vi "ReadDispenseCount (SubVI).vi"(10 "Base Path":path) -> (2 "appended array":i32[](array[numeric]))   [LabVIEW 2013]
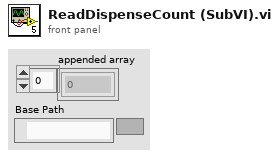
[diagram p1: front panel]
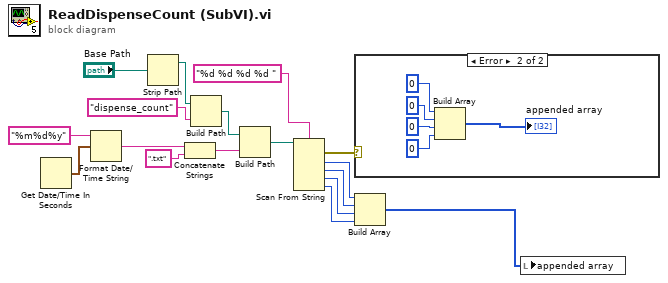
[diagram p0: block diagram]
diagram:
  n1 = Get Date/Time In Seconds() -> (seconds since 1Jan1904=w12:timestamp)
  n2 = Format Date/Time String(time format string (%c)="%m%d%y", seconds (now)=w12) -> (date/time string=w10:string)  [unwired: 1 in]
  n3 = Strip Path(path="Base Path") -> (stripped path=w14:path)  [unwired: 1 out]
  n4 = Concatenate Strings(w10, ".txt" ("string")) -> (w8:string)
  n5 = Build Path(base path=w14, name or relative path="dispense_count") -> (appended path=w17:path)
  n6 = Build Path(base path=w17, name or relative path=w8) -> (appended path=w7:path)
  n7 = Scan From String("%d %d %d %d " ("format string"), w7) -> (w15:errorcluster, output 1=w2:i32, output 2=w5:i32, output 3=w4:i32, output 4=w3:i32)  [unwired: 5 in, 1 out]
  n8 = case shown="Error" w15 {
    frame No Error {
    }
    frame Error {
      n9 = Build Array(0 ("element"), 0 ("element"), 0 ("element"), 0 ("element")) -> (→"appended array":i32[])
    }
  }
  n10 = Build Array(w2, w5, w4, w3) -> (w1:i32[])
  n11 = local write "appended array"(w1) -> ()
